vi "Fetch Model Config.vi"(8 "error in (no error)":errorcluster, 10 "SQL Query":string, 11 "Refnum in":T3) -> (0 "error out":errorcluster, 2 "Hardware Settings Cluster":T1={"Sensor ID *"=0, "Target Sample Rate (Hz) *"=1000.0, "Steady-State Duration (s) *"=5, "Allowed Tolerance (%) FS *"=0.5, "Max Settling Timeout (s) *"=5, "Physical Channel"="", "Measurement Role"=enum."Controller"}, 3 "Refnum out":T3)   [LabVIEW 2026, in "Database.lvlib"]
uses:
  Database.lvlib
  <vilib>/addons/database/Connection.llb/Conn ObjectReference.ctl
  Acquisition/Instrument Specifications Cluster Configuration.ctl
  controls/UI/Measurement Role.ctl
  controls/Messaging Payloads/Processed Calibration Point.ctl
  controls/UI/Direction.ctl
  Processing/Test Status.ctl
  <vilib>/addons/database/Connection.llb/Conn Execute.vi
  <vilib>/addons/database/Recordset.llb/Rec Fetch Double Data (R).vi
  <vilib>/addons/database/Recordset.llb/Rec Fetch Integer Data (R).vi
  <vilib>/addons/database/Recordset.llb/Rec Destroy - Connection.vi
  <vilib>/addons/database/NI_Database_API.lvlib
  Acquisition/Acquisition.lvlib
  Settings/Settings.lvlib
  Analysis/Analysis.lvlib
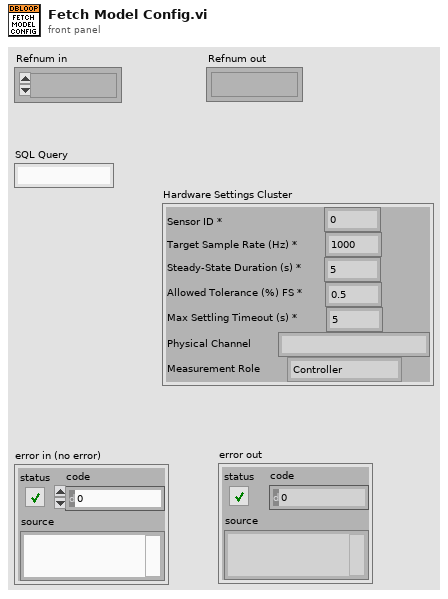
[diagram p1: front panel]
types:
  T1 = typedef "Acquisition.lvlib/Instrument Specifications Cluster Configuration.ctl" = cluster{"Sensor ID *":i32, "Target Sample Rate (Hz) *":dbl, "Steady-State Duration (s) *":i32, "Allowed Tolerance (%) FS *":dbl, "Max Settling Timeout (s) *":i32, "Physical Channel":string, "Measurement Role":T2}
  T2 = typedef "Settings.lvlib/Measurement Role.ctl" = enum16{"Controller", "Reference", "UUT", "Disable", "All"}
  T3 = typedef "NI_Database_API.lvlib/Conn ObjectReference.ctl" = refnum<k1>
  T4 = typedef "Processed Calibration Point.ctl" = cluster{"Reference Value":dbl, "Measured Value":dbl, "Error":dbl, "Pass/Fail":bool, "Setpoint":dbl, "Cycle Number":i32, "Direction":T5, "Test Status":T6}
  T5 = typedef "Settings.lvlib/Direction.ctl" = enum16{"Acsending", "Descending"}
  T6 = typedef "Analysis.lvlib/Test Status.ctl" = enum16{"Overall Pass", "Overall Fail", "Test Running"}
  T7 = typedef "NI_Database_API.lvlib/Rec ObjectReference.ctl" = refnum<k1>
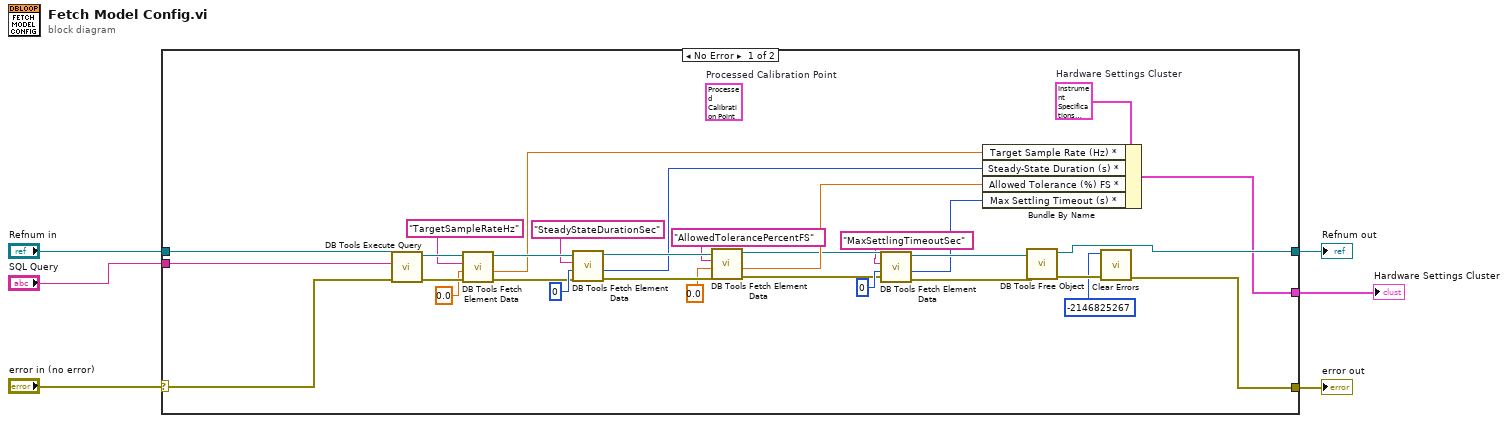
[diagram p0: block diagram]
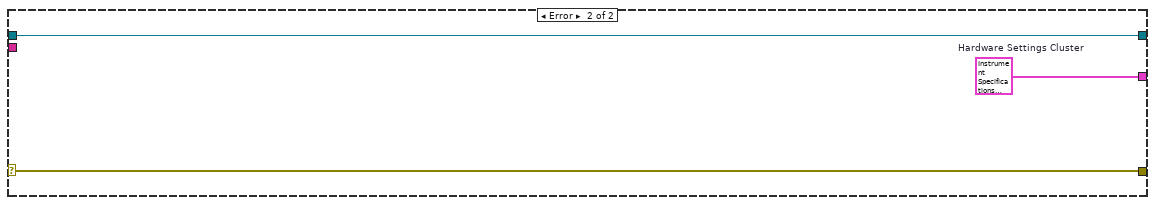
[diagram p2: hidden frame]
diagram:
  n1 = case shown="No Error" "error in (no error)" {
    selector: "error in (no error)" -> [w15 w40]
    tunnel: [w37 w39] -> w6
    tunnel: [w36 w40] -> w5
    tunnel: [w31 w38] -> w1
    tunnel: "SQL Query" -> [w30 _]
    tunnel: "Refnum in" -> [w29 w39]
    frame No Error {
      (unwired) T4 {"Reference Value"=0.0, "Measured Value"=0.0, "Error"=0.0, "Pass/Fail"=FALSE, "Setpoint"=0.0, "Cycle Number"=0, "Direction"=enum."Acsending", "Test Status"=enum."Overall Pass"}  # Processed Calibration Point
      w14 = T1 {"Sensor ID *"=0, "Target Sample Rate (Hz) *"=1000.0, "Steady-State Duration (s) *"=5, "Allowed Tolerance (%) FS *"=0.5, "Max Settling Timeout (s) *"=5, "Physical Channel"="", "Measurement Role"=enum."Controller"}  # Hardware Settings Cluster
      n2 = call-poly <vilib>:"DB Tools Execute Query.vi"("error in (no error)"=w15, "SQL query"=w30, "connection reference"=w29) -> ("error out"=w34:errorcluster, "recordset reference"=w33:T7)  [unwired: 5 in]
      n3 = call-poly <vilib>:"DB Tools Fetch Element Data.vi"("error in (no error)"=w34, "type"=0.0, "column index"="TargetSampleRateHz", "recordset reference"=w33) -> ("error out"=w21:errorcluster, "data"=w18:dbl, "recordset reference out"=w20:T7)  [unwired: 3 in]
      n4 = call-poly <vilib>:"DB Tools Fetch Element Data.vi"("error in (no error)"=w21, "type"=0, "column index"="SteadyStateDurationSec", "recordset reference"=w20) -> ("error out"=w26:errorcluster, "data"=w23:i32, "recordset reference out"=w27:T7)  [unwired: 3 in]
      n5 = call-poly <vilib>:"DB Tools Fetch Element Data.vi"("error in (no error)"=w26, "type"=0.0, "column index"="AllowedTolerancePercentFS", "recordset reference"=w27) -> ("error out"=w12:errorcluster, "data"=w28:dbl, "recordset reference out"=w10:T7)  [unwired: 3 in]
      n6 = call-poly <vilib>:"DB Tools Fetch Element Data.vi"("error in (no error)"=w12, "type"=0, "column index"="MaxSettlingTimeoutSec", "recordset reference"=w10) -> ("error out"=w11:errorcluster, "data"=w8:i32, "recordset reference out"=w9:T7)  [unwired: 3 in]
      n7 = Bundle By Name(cluster=w14, "Target Sample Rate (Hz) *"=w18, "Steady-State Duration (s) *"=w23, "Allowed Tolerance (%) FS *"=w28, "Max Settling Timeout (s) *"=w8) -> (w31:T1)
      n8 = call-poly <vilib>:"DB Tools Free Object.vi"("error in (no error)"=w11, "recordset reference"=w9) -> ("error out"=w35:errorcluster, "connection reference"=w37:T3)  [unwired: 8 in]
      n9 = call <vilib>:"Clear Errors.vi"("error in (no error)"=w35, "specific error code to clear (0: all)"=-2146825267) -> ("error out"=w36:errorcluster)  [unwired: 4 in, 1 out]
    }
    frame Error {
      w38 = T1 {"Sensor ID *"=0, "Target Sample Rate (Hz) *"=1000.0, "Steady-State Duration (s) *"=5, "Allowed Tolerance (%) FS *"=0.5, "Max Settling Timeout (s) *"=5, "Physical Channel"="", "Measurement Role"=enum."Controller"}  # Hardware Settings Cluster
    }
  }
  "Refnum out" <- w6
  "error out" <- w5
  "Hardware Settings Cluster" <- w1
